vi "FlatToRichniswitch_grpc_CloseRequest.vi"(5 "OutputClusterType":T1, 11 "InputCluster":T3) -> (3 "OutputCluster":T1)   [LabVIEW 2021, in "NI Switch Client.lvlib"]
uses:
  NI Switch Client.lvlib
  nidevice_grpc_Session_session/nidevice_grpc_Session_session.lvclass
  nidevice_grpc_Session.ctl
  niswitch_grpc_CloseRequest.ctl
  nidevice_grpc_Session_Flat.ctl
  niswitch_grpc_CloseRequest_Flat.ctl
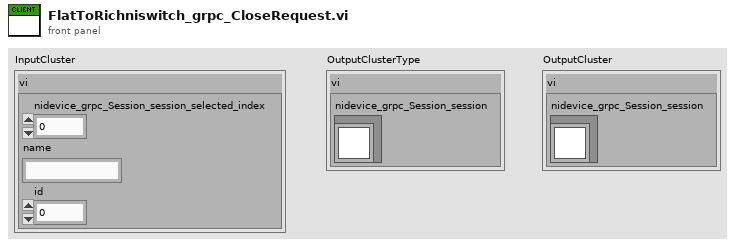
[diagram p1: front panel]
types:
  T1 = typedef "NI Switch Client.lvlib/niswitch_grpc_CloseRequest.ctl" = cluster{"vi":T2}
  T2 = typedef "NI Switch Client.lvlib/nidevice_grpc_Session.ctl" = cluster{"nidevice_grpc_Session_session":refnum<class "nidevice_grpc_Session_session.lvclass">}
  T3 = typedef "NI Switch Client.lvlib/niswitch_grpc_CloseRequest_Flat.ctl" = cluster{"vi":T4}
  T4 = typedef "NI Switch Client.lvlib/nidevice_grpc_Session_Flat.ctl" = cluster{"nidevice_grpc_Session_session_selected_index":i32, "name":string, "id":u32}
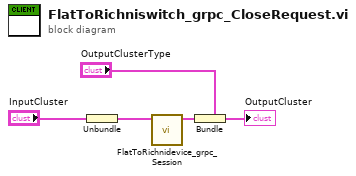
[diagram p0: block diagram]
diagram:
  n1 = Unbundle "Unbundle"("InputCluster") -> ("vi"=w2:T4)
  n2 = call "FlatToRichnidevice_grpc_Session.vi"("InputCluster"=w2) -> ("OutputCluster"=w1:T2)  [unwired: 10 in]
  n3 = Bundle "Bundle"(cluster="OutputClusterType", "vi"=w1) -> (→"OutputCluster":T1)
